vi "Build DMA Channel Dictionary.vi"(8 "error in (no error)":errorcluster, 11 "old bitfile dma channels":T1[](array[typedef]) {"Data Type" format="%.0x"}) -> (0 "error out":errorcluster, 3 "scalar channels dictionary":variant)   [LabVIEW 2020, in "FPGA Addon System Explorer.lvlib"]
uses:
  FPGA Addon System Explorer.lvlib
  Addon Shared/Types/DMA Information.ctl
  Addon Shared/Types/FPGA Addon Data Type.ctl
  Addon Shared/FPGA Addon Shared.lvlib
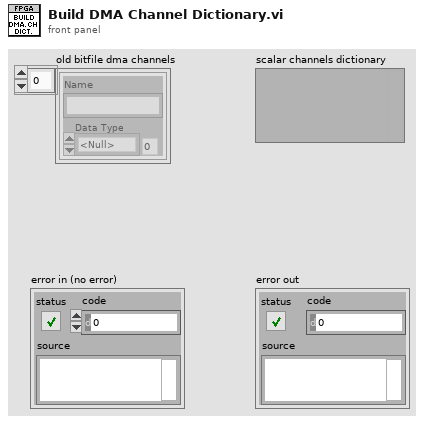
[diagram p1: front panel]
types:
  T1 = typedef "FPGA Addon Shared.lvlib/DMA Information.ctl" = cluster{"Name":string, "Data Type":T2}
  T2 = typedef "FPGA Addon Shared.lvlib/FPGA Addon Data Type.ctl" = enum8{"<Null>", "I8", "I16", "I32", "I64", "U8", "U16", "U32", "U64", "SGL", "Boolean", "Analog PWM In Settings", "Analog PWM In", "Digital PWM In Settings", "Digital PWM In", "Digital PWM Out", "Sine Out", "FXP", "FXP+/-24.5", "FXP+/-16.5", "FXP+/-32.8", "FXP+/-64.32", "FXP+/-16.7", "FXP+/-20.5", "FXP+/-27.5", "FXP+/-32.16", "FXP+16.3", "FXP+18.3", "Digital Static In", "Digital Static Out", "Digital Static In Settings", "Digital WSS Out", "Quad Encoder Settings", "Quad Encoder In", "Group"}
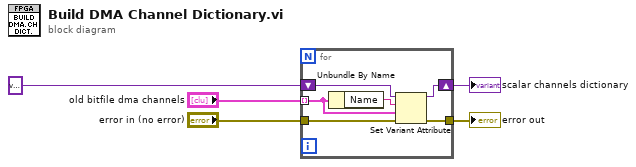
[diagram p0: block diagram]
diagram:
  n1 = for {
    tunnel: "old bitfile dma channels" -> [w8] mode=indexing
    tunnel: "error in (no error)" -> [w10]
    tunnel: [w9] -> w5
    shift-right: [w6] -> w4
    shift-left: variant -> [w7]
    n2 = Unbundle By Name(w8) -> ("Name"=w11:string)
    n3 = Set Variant Attribute(Variant=w7, name=w11, value=w8, error in=w10) -> (Variant out=w6:variant, error out=w9:errorcluster)  [unwired: 1 out]
  }
  "error out" <- w5
  "scalar channels dictionary" <- w4
